vi "DoPurge.vi"(8 "error in (no error)":errorcluster, 11 "Graph in":cluster{dbl[], dbl[]}) -> (0 "error out":errorcluster, 2 "StabilityAchieved":bool, 3 "Values":cluster{dbl[], dbl[]})   [LabVIEW 2013]
uses:
  GlobalVariables/ValveParameters.vi
  GlobalVariables/PressureAndTimeSamples.vi
  GlobalVariables/StabilizationSettings.vi
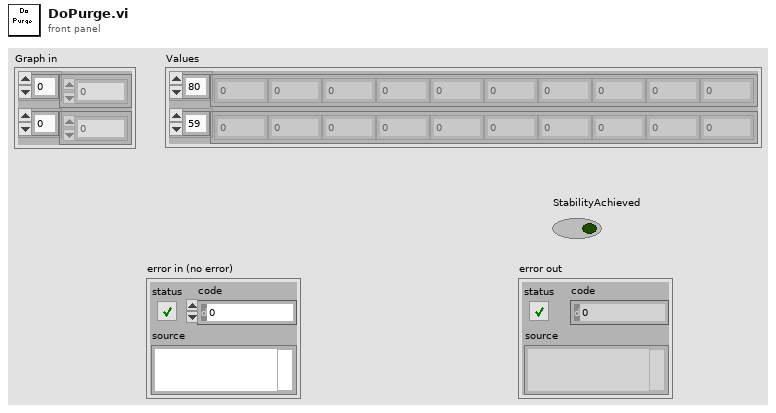
[diagram p1: front panel]
types:
  T1 = cluster{"baudrate":u32, "databits":u16, "paritybit":u16, "stopbits":u16, "flux control":u16, "Port":string, "Serial Parameters":cluster{"Mode":enum16{"RTU", "ASCII"}, "Slave Address":u8}, "Timeout":u32, "Valve mapping":cluster{"Inlet Valve":u8, "V1":u8, "V2":u8, "Sample Valve":u8, "Outlet Valve":u8}}
  T2 = cluster{"MinimalWaitTime":u32, "VarianceTrigger":dbl, "MaxWaitTime":u32}
  T3 = cluster{"TimeSamples":dbl[], "PressureSamples":dbl[]}
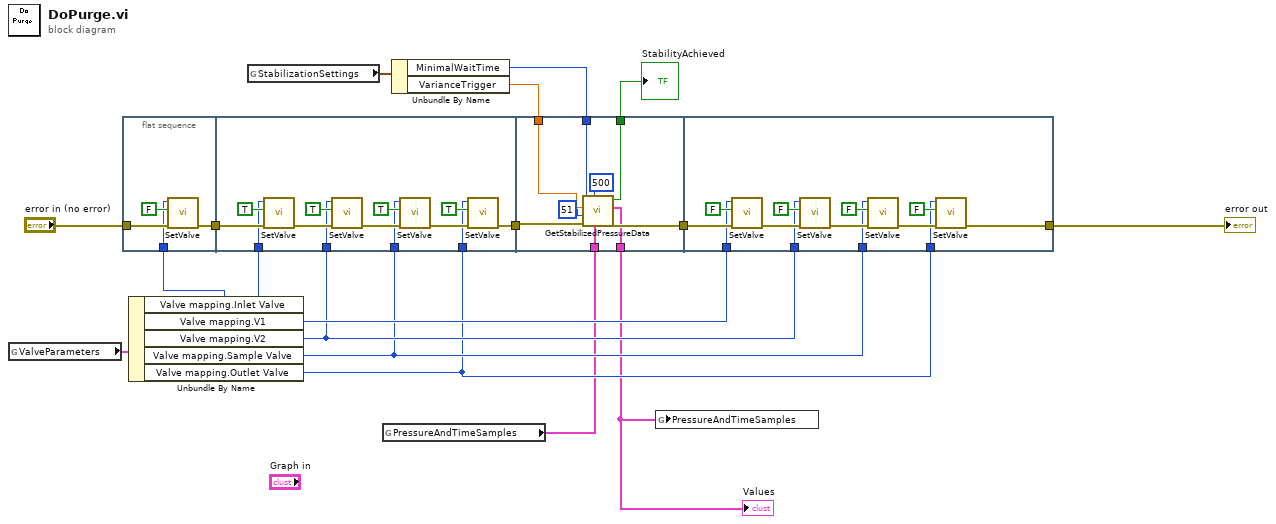
[diagram p0: block diagram]
diagram:
  n1 = global read "ValveParameters.vi" "ValveParameters"() -> (w14:T1)
  n2 = flat-sequence {
    tunnel: [w20] -> w8
    tunnel: "error in (no error)" -> [w19]
    tunnel: w13 -> [w18]
    tunnel: w8 -> [w31]
    tunnel: [w26] -> w15
    tunnel: w12 -> [w25]
    tunnel: w11 -> [w24]
    tunnel: w10 -> [w23]
    tunnel: w9 -> [w22]
    tunnel: w15 -> [w42]
    tunnel: [w43] -> w7
    tunnel: w6 -> [w41]
    tunnel: [w40] -> w5
    tunnel: w3 -> [w37]
    tunnel: w2 -> [w36]
    tunnel: [w35] -> w1
    tunnel: [w44] -> w16
    tunnel: w12 -> [w48]
    tunnel: w11 -> [w47]
    tunnel: w10 -> [w46]
    tunnel: w9 -> [w45]
    tunnel: w7 -> [w52]
    frame #0 {
      n3 = call "SetValve.vi"("error in"=w19, "ON"=FALSE, "Valve"=w18) -> ("error out"=w20:errorcluster)  [unwired: 8 in]
    }
    frame #1 {
      n4 = call "SetValve.vi"("error in"=w31, "ON"=TRUE, "Valve"=w25) -> ("error out"=w32:errorcluster)  [unwired: 8 in]
      n5 = call "SetValve.vi"("error in"=w32, "ON"=TRUE, "Valve"=w24) -> ("error out"=w33:errorcluster)  [unwired: 8 in]
      n6 = call "SetValve.vi"("error in"=w33, "ON"=TRUE, "Valve"=w23) -> ("error out"=w34:errorcluster)  [unwired: 8 in]
      n7 = call "SetValve.vi"("error in"=w34, "ON"=TRUE, "Valve"=w22) -> ("error out"=w26:errorcluster)  [unwired: 8 in]
    }
    frame #2 {
      n8 = call "GetStabilizedPressureData.vi"("Graph in"=w41, "WaitTime"=500, "error in"=w42, "SampleCount"=51, "Variance/Mean Trigger"=w37, "MinimalWaitTimems"=w36) -> ("error out"=w43:errorcluster, "Values"=w40:cluster{dbl[], dbl[]}, "StabilityAchieved"=w35:bool)  [unwired: 3 in]
    }
    frame #3 {
      n9 = call "SetValve.vi"("error in"=w52, "ON"=FALSE, "Valve"=w48) -> ("error out"=w51:errorcluster)  [unwired: 8 in]
      n10 = call "SetValve.vi"("error in"=w51, "ON"=FALSE, "Valve"=w47) -> ("error out"=w50:errorcluster)  [unwired: 8 in]
      n11 = call "SetValve.vi"("error in"=w50, "ON"=FALSE, "Valve"=w46) -> ("error out"=w49:errorcluster)  [unwired: 8 in]
      n12 = call "SetValve.vi"("error in"=w49, "ON"=FALSE, "Valve"=w45) -> ("error out"=w44:errorcluster)  [unwired: 8 in]
    }
  }
  n13 = Unbundle By Name(w14) -> ("Valve mapping.Inlet Valve"=w13:u8, "Valve mapping.V1"=w12:u8, "Valve mapping.V2"=w11:u8, "Valve mapping.Sample Valve"=w10:u8, "Valve mapping.Outlet Valve"=w9:u8)
  n14 = global read "StabilizationSettings.vi" "StabilizationSettings"() -> (w4:T2)
  n15 = global read "PressureAndTimeSamples.vi" "PressureAndTimeSamples"() -> (w6:T3)
  n16 = Unbundle By Name(w4) -> ("MinimalWaitTime"=w2:u32, "VarianceTrigger"=w3:dbl)
  n17 = global write "PressureAndTimeSamples.vi" "PressureAndTimeSamples"(w5) -> ()
  "error out" <- w16
  "Values" <- w5
  "StabilityAchieved" <- w1
